vi "File Save Header to FA File.vi"(6 "BPM and PS selection":T1, 7 "Acquisition period (us)":u32, 8 "error in (no error)":errorcluster, 9 "PS Reading Names":string[](array[string]), 10 "BPM Reading Names":string[](array[string]), 11 "FA File Reference":refnum<file>) -> (0 "error out":errorcluster)   [LabVIEW 2011, in "File VIs.lvlib"]
uses:
  Types Definitions/Type BPM and PS select cluster.ctl
  File VIs.lvlib
  Type Definitions.lvlib
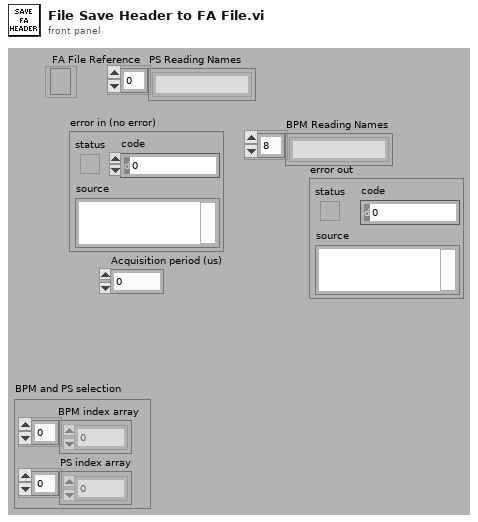
[diagram p1: front panel]
types:
  T1 = typedef "Type Definitions.lvlib/Type BPM and PS select cluster.ctl" = cluster{"BPM index array":u32[], "PS index array ":u32[]}
  T2 = enum16{"big-endian, network order", "native, host order", "little-endian"}
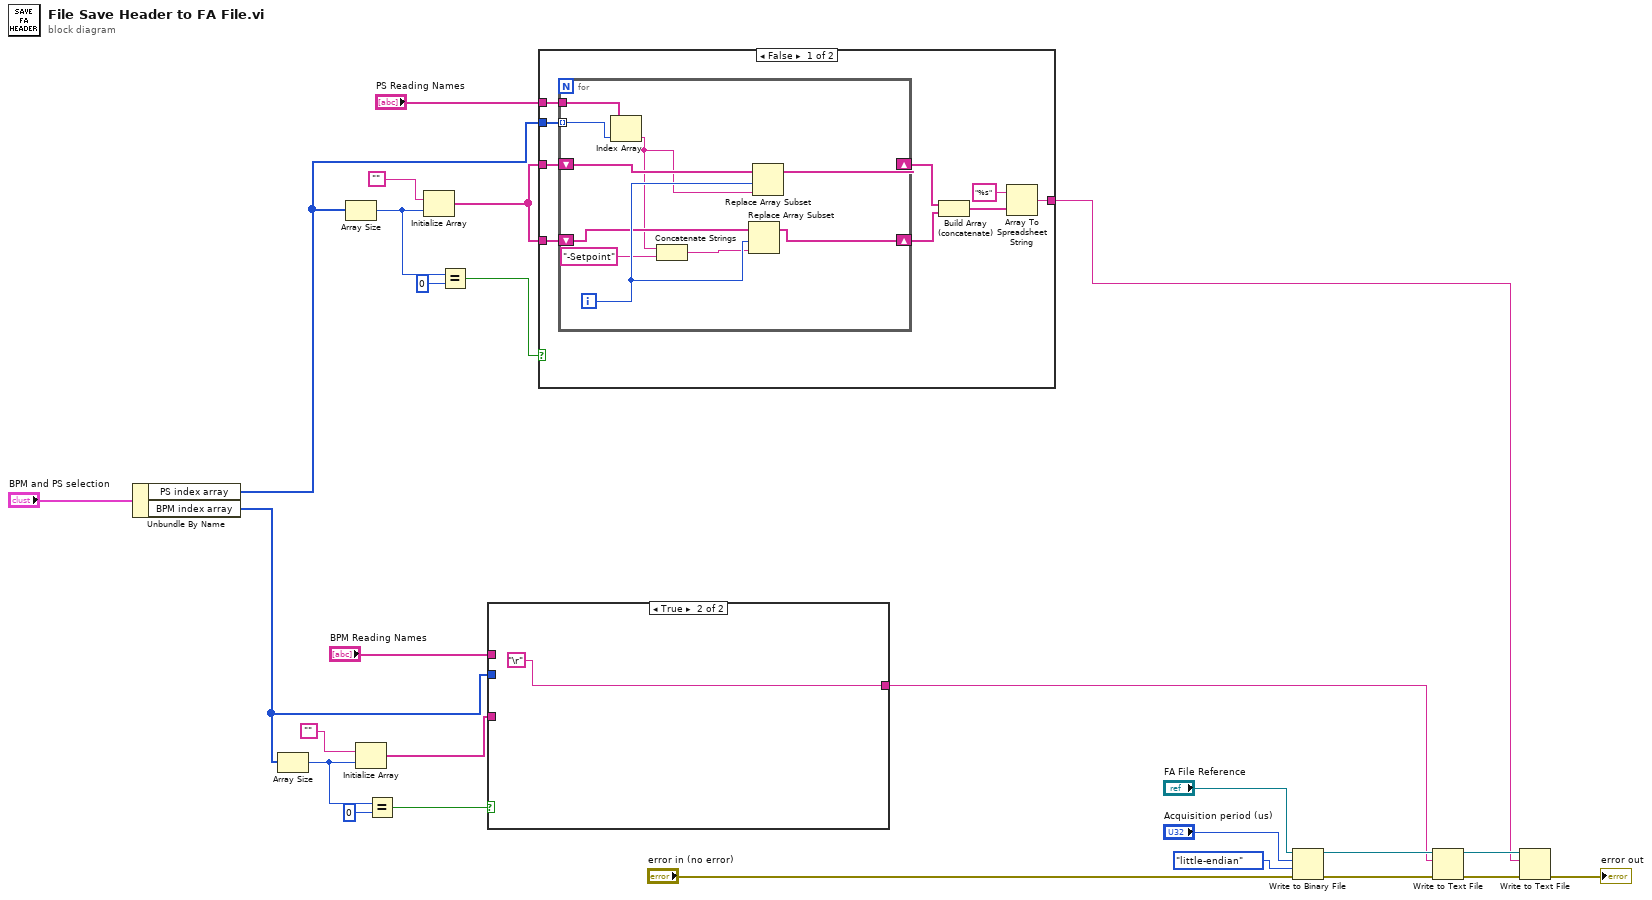
[diagram p0: block diagram]
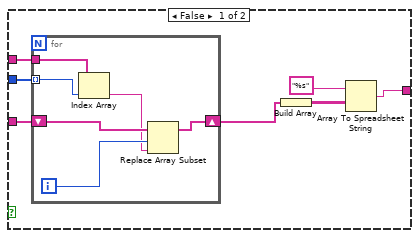
[diagram p2: hidden frame]
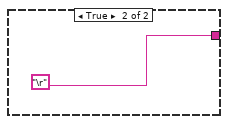
[diagram p3: hidden frame]
diagram:
  n1 = Unbundle By Name("BPM and PS selection") -> ("PS index array"=w3:u32[], "BPM index array"=w14:u32[])
  n2 = Array Size(array=w14) -> (size(s)=w12:i32)
  n3 = Array Size(array=w3) -> (size(s)=w7:i32)
  n4 = Initialize Array("", w12) -> (w15:string[])
  n5 = Equal?(x=w12, y=0) -> (x = y?=w10:bool)
  n6 = Initialize Array("", w7) -> (w5:string[])
  n7 = Equal?(x=w7, y=0) -> (x = y?=w4:bool)
  n8 = case shown="True" w10 {
    tunnel: "BPM Reading Names" -> [w33 _]
    tunnel: w14 -> [w32 _]
    tunnel: w15 -> [w31 _]
    tunnel: [w27 "\r"] -> w1
    frame False {
      n9 = for {
        tunnel: w33 -> [w35]
        tunnel: w32 -> [w36] mode=indexing
        shift-right: [w37] -> w29
        shift-left: w31 -> [w39]
        i -> [w38]
        n10 = Index Array(array=w35, index=w36) -> (element=w34:string)
        n11 = Replace Array Subset(array=w39, new element=w34, index=w38) -> (w37:string[])
      }
      n12 = Build Array(w29) -> (w28:string[][])
      n13 = Array To Spreadsheet String(array=w28, 3:"%s" ("format string")) -> (spreadsheet string=w27:string)  [unwired: 1 in]
    }
    frame True {
    }
  }
  n14 = case shown="False" w4 {
    tunnel: "PS Reading Names" -> [w49 _]
    tunnel: w3 -> [w48 _]
    tunnel: w5 -> [w47 _]
    tunnel: w5 -> [w46 _]
    tunnel: [w41 "\r"] -> w2
    frame False {
      n15 = for {
        tunnel: w49 -> [w56]
        tunnel: w48 -> [w57] mode=indexing
        shift-right: [w58] -> w43
        shift-left: w47 -> [w59]
        shift-right: [w55] -> w42
        shift-left: w46 -> [w53]
        i -> [w54]
        n16 = Index Array(array=w56, index=w57) -> (element=w50:string)
        n17 = Concatenate Strings(w50, "-Setpoint") -> (w52:string)
        n18 = Replace Array Subset(array=w53, new element=w52, index=w54) -> (w55:string[])
        n19 = Replace Array Subset(array=w59, new element=w50, index=w54) -> (w58:string[])
      }
      n20 = Build Array (concatenate)(w43, w42) -> (w45:string[])
      n21 = Array To Spreadsheet String(array=w45, 3:"%s" ("format string")) -> (spreadsheet string=w41:string)  [unwired: 1 in]
    }
    frame True {
    }
  }
  n22 = Write to Binary File(file (use dialog)="FA File Reference", data="Acquisition period (us)", error in="error in (no error)", 9:T2."little-endian" ("byte order (0:big-endian, network order)")) -> (refnum out=w21:refnum<file>, error out=w19:errorcluster)  [unwired: 2 in, 1 out]
  n23 = Write to Text File(file (use dialog)=w21, text=w1, error in=w19) -> (refnum out=w25:refnum<file>, error out=w26:errorcluster)  [unwired: 1 in, 1 out]
  n24 = Write to Text File(file (use dialog)=w25, text=w2, error in=w26) -> (error out=→"error out":errorcluster)  [unwired: 1 in, 2 out]
